vi "Speak withDPO-4034 (SUBVI).vi"(2 "Send Command":string, 3 "Send:  TRUE\nRecive: FALSE":bool, 4 "VISA Resource Name":refnum<visa-resource-name>) -> (0 "Read Buffer":string)   [LabVIEW 2010]
panel:
  out "error out":errorcluster
  # "RECALL:SETUP \"D:\\ABM\\ABMconfigureAutomatict.set\""
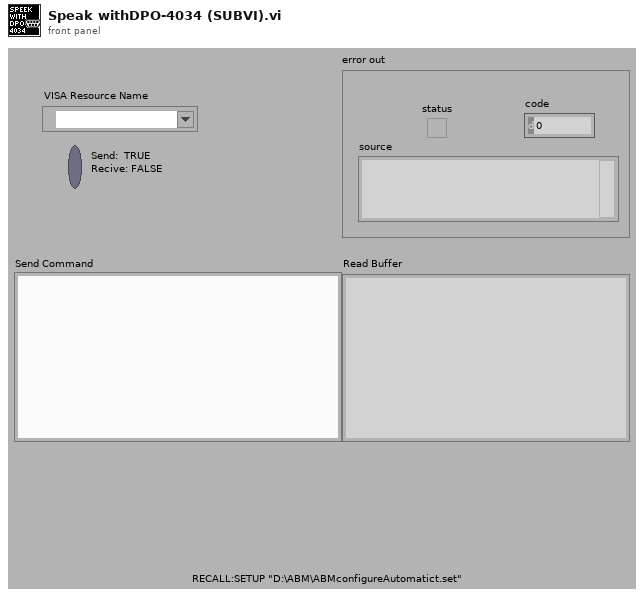
[diagram p1: front panel]
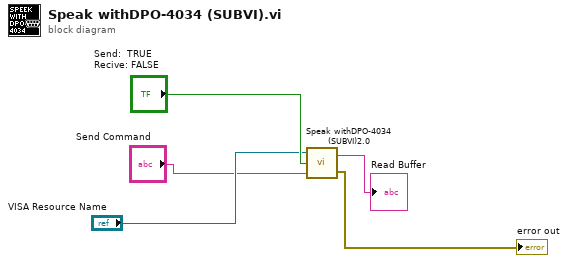
[diagram p0: block diagram]
diagram:
  n1 = call "Speak withDPO-4034 (SUBVI)2.0.vi"("Send Command"="Send Command", "Send:  TRUE\nRecive: FALSE"="Send:  TRUE\nRecive: FALSE", "VISA Resource Name"="VISA Resource Name") -> ("error out"=→"error out":errorcluster, "Read Buffer"=→"Read Buffer":string)
